vi "Roller Teleop Inputs.vi"(8 "error in (no error)":errorcluster) -> (0 "error out":errorcluster, 2 "Roller Input Data":T1)   [LabVIEW 2014]
uses:
  Roller Input Data.ctl
  Robot Global Data.vi
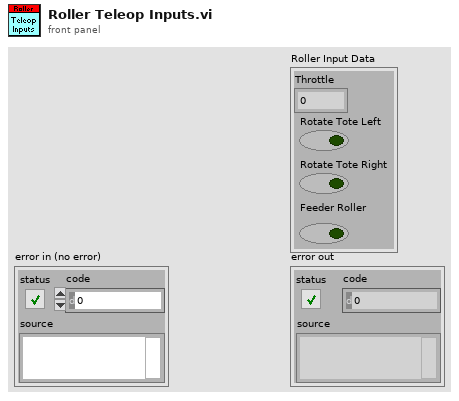
[diagram p1: front panel]
types:
  T1 = typedef "Roller Input Data.ctl" = cluster{"Throttle":dbl, "Rotate Tote Left":bool, "Rotate Tote Right":bool, "Feeder Roller":bool}
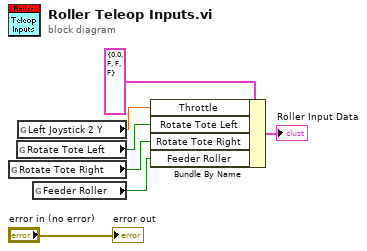
[diagram p0: block diagram]
diagram:
  n1 = global read "Robot Global Data.vi" "Rotate Tote Right"() -> (w3:bool)
  n2 = global read "Robot Global Data.vi" "Rotate Tote Left"() -> (w4:bool)
  n3 = global read "Robot Global Data.vi" "Left Joystick 2 Y"() -> (w5:dbl)
  n4 = global read "Robot Global Data.vi" "Feeder Roller"() -> (w1:bool)
  n5 = Bundle By Name(cluster=T1 {"Throttle"=0.0, "Rotate Tote Left"=FALSE, "Rotate Tote Right"=FALSE, "Feeder Roller"=FALSE} ("Roller Input Data"), "Throttle"=w5, "Rotate Tote Left"=w4, "Rotate Tote Right"=w3, "Feeder Roller"=w1) -> (→"Roller Input Data":T1)
  "error out" <- "error in (no error)"
